vi "3dShit.vi"() -> ()   [LabVIEW 2021]
uses:
  <vilib>/Math Plots/3D Math Plots/3D Surface/3D Surface XCtrl/3D Surface.xctl
  <vilib>/Utility/file.llb/Read Delimited Spreadsheet (DBL).vi
  <vilib>/Analysis/NI_AALPro.lvlib
  <vilib>/Analysis/6fits.llb/nD B-Spline Fit.vi
  <vilib>/Math Plots/3D Math Plots/3D Surface/3D Surface Datatype/3D Surface Datatype.lvclass
  <vilib>/Math Plots/3D Math Plots/3D Surface/3D Surface Datatype/Public/Plot Helper (Matrix).vi
panel:
  in  "Slide":cluster{dbl, dbl, dbl, dbl, dbl, dbl}(slide)={248.76658476658477, 249.17936117936117, 312.74692874692875, 365.58230958230956, 381.26781326781327, 224.0} scale=224.0..392.0
  out "min value":dbl
  out "max value":dbl
  in  "Array":dbl[](array[numeric])
  out "3D Surface":refnum<class "3D Plot Datatype.lvclass">[](xcontrol)
  out "size(s)":i32[](array[numeric])
  out "Waveform Graph":dbl[][](graph)
  in  "Custom Marker Colors":u32[](array[colorbox])=[15663322, 786687, 9567230, 6618880, 16774656, 16757546, 16711680]
  in  "stop":bool
  out "Surface CV Plot":dbl[][](graph)
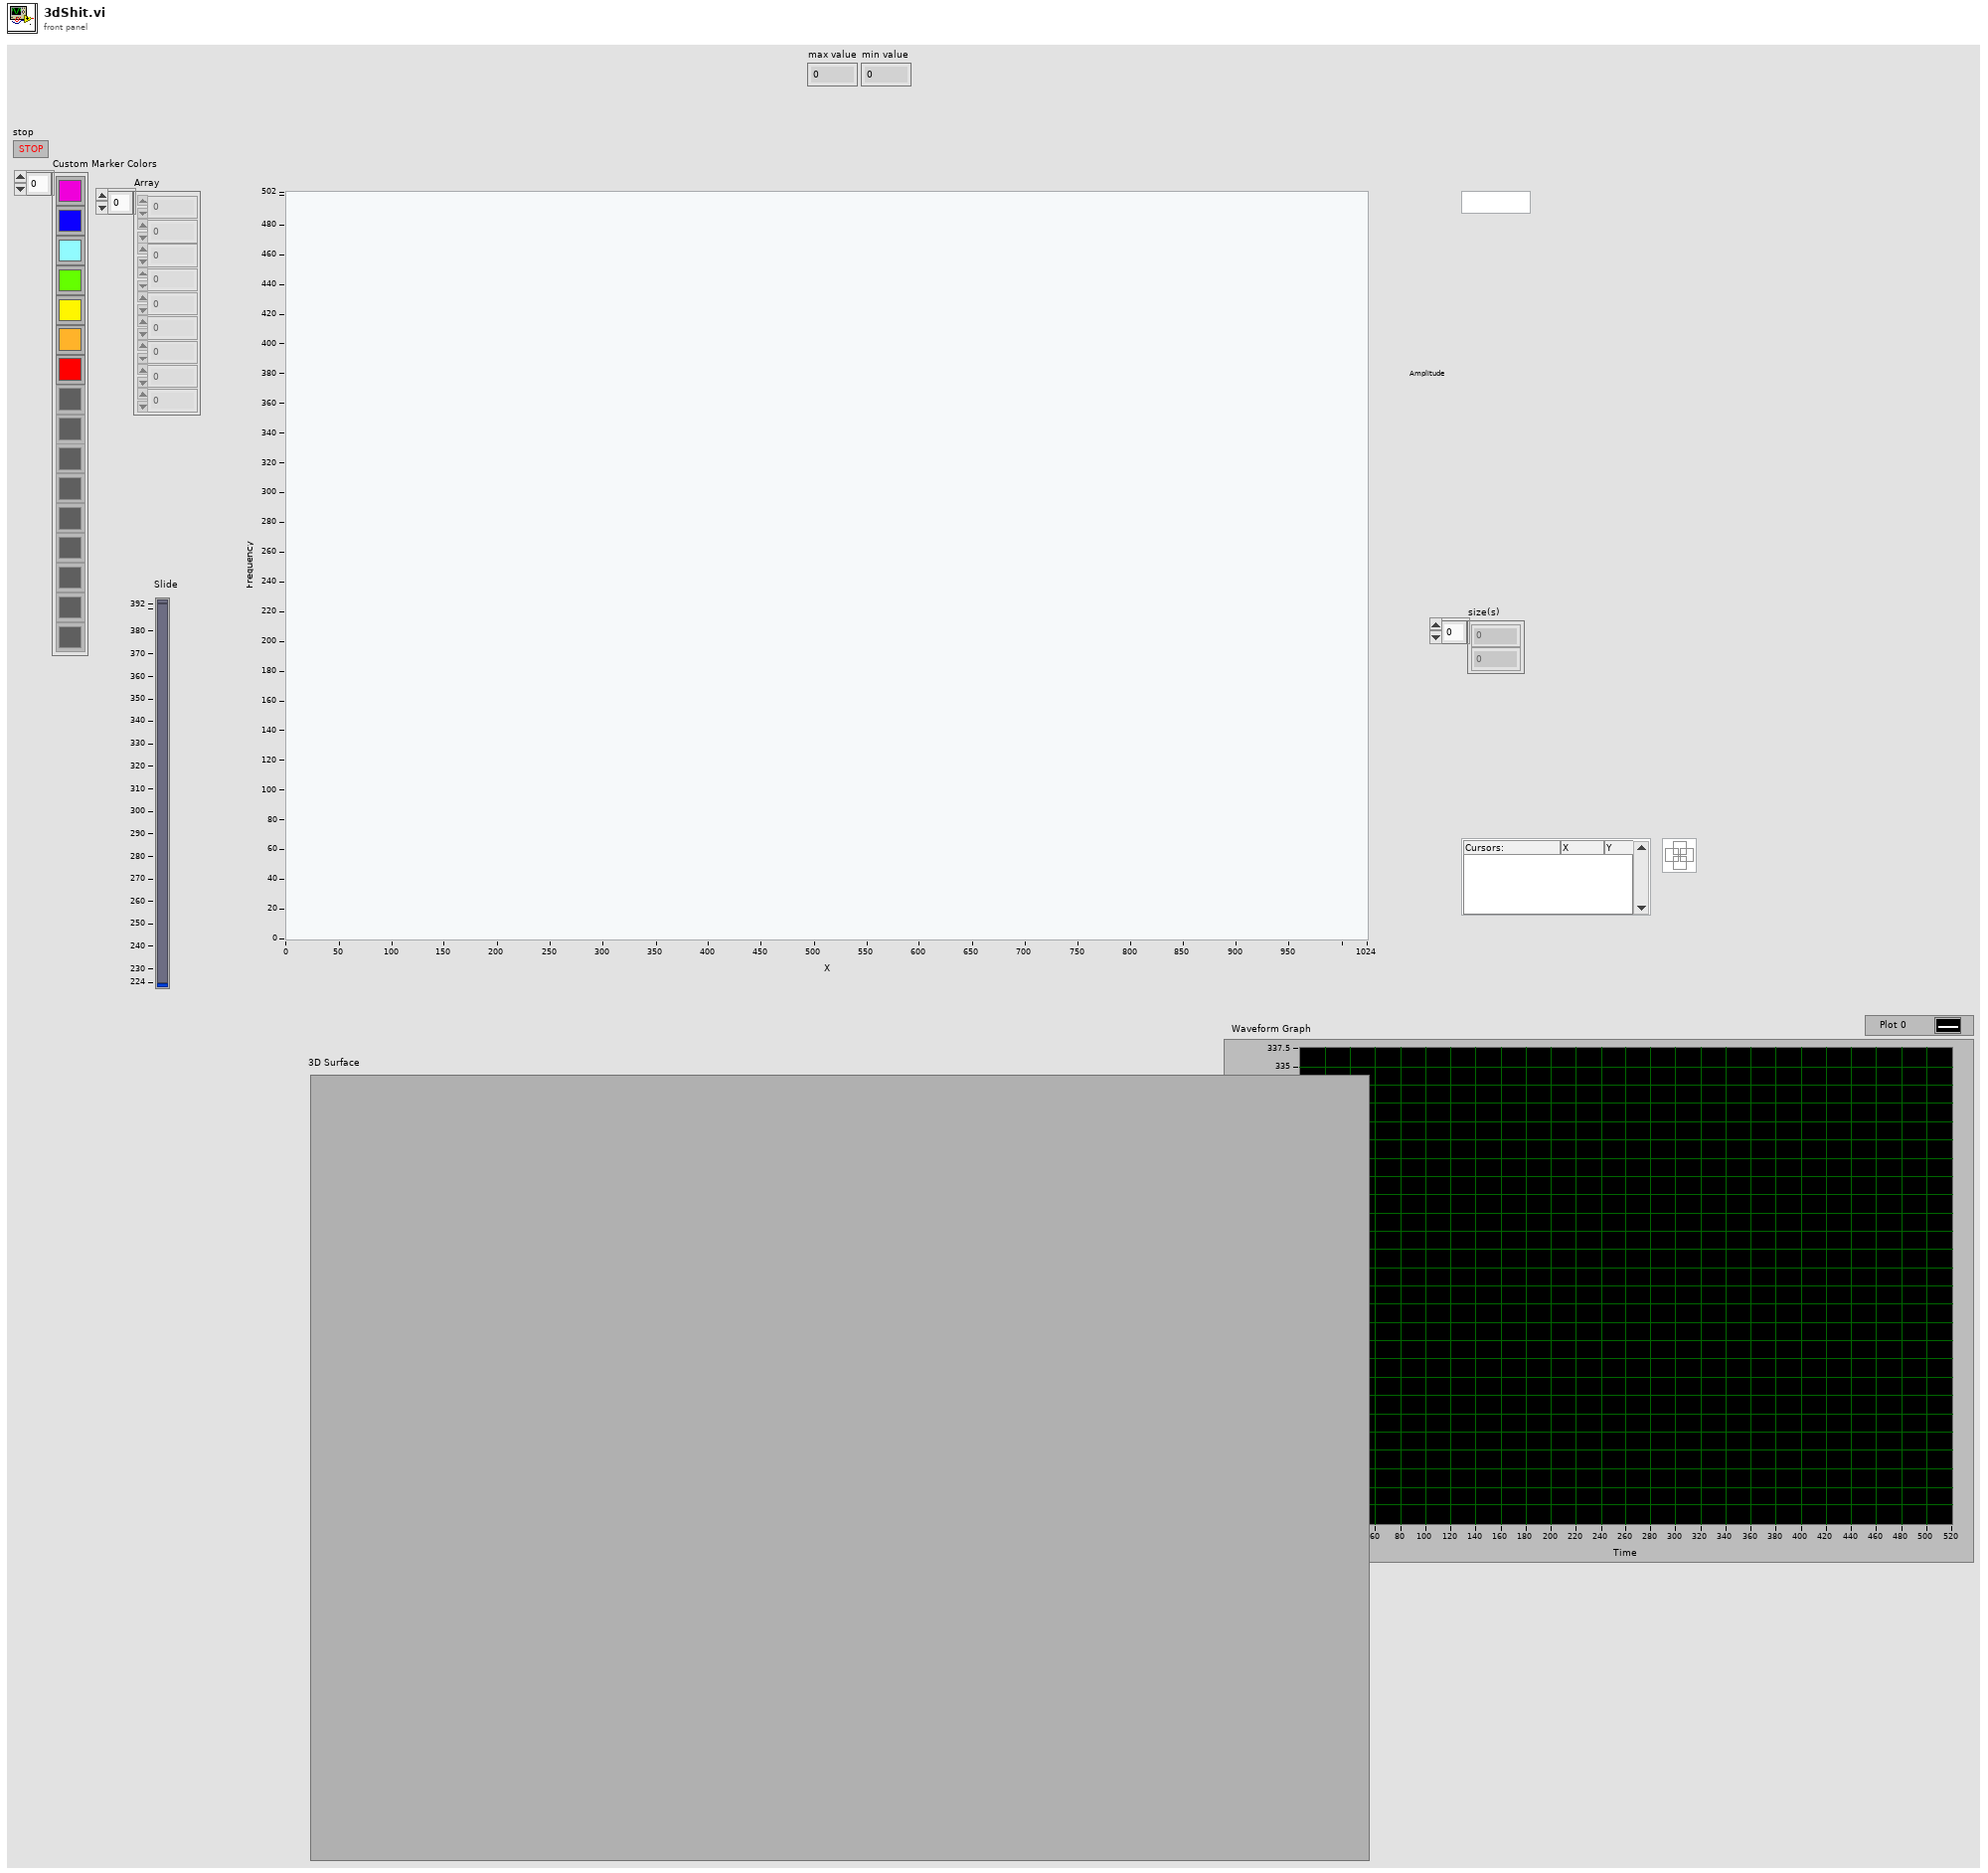
[diagram p1: front panel]
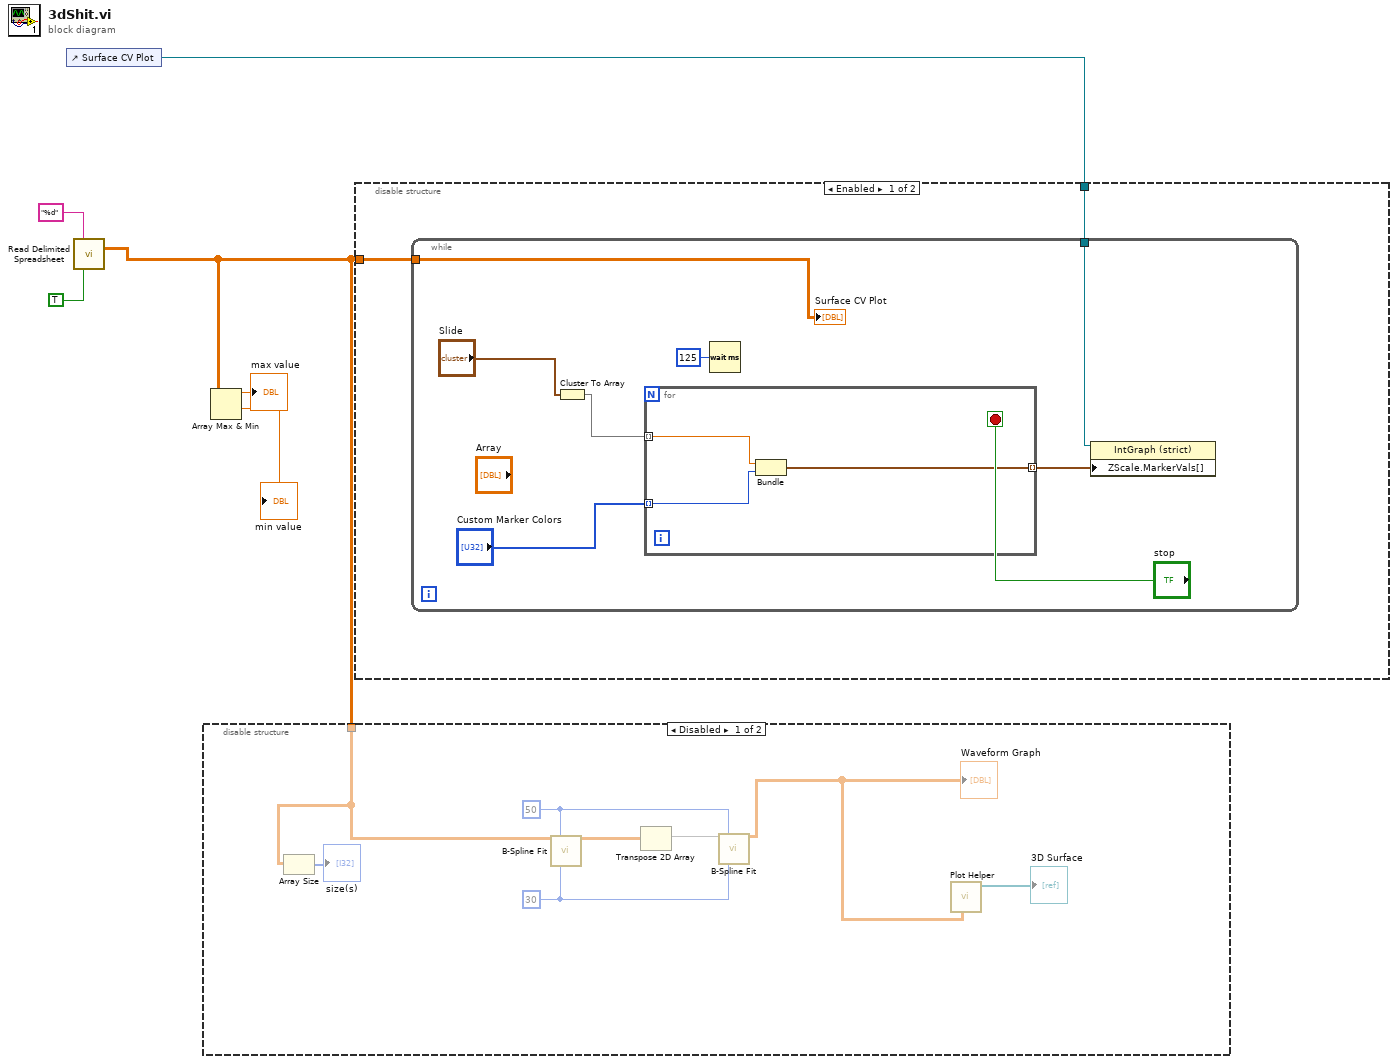
[diagram p0: block diagram]
diagram:
  n1 = control-ref of="Surface CV Plot"() -> (w4:refnum<vi>)
  n2 = call-poly <vilib>:"Read Delimited Spreadsheet.vi"("format (%.3f)"="%d", "transpose? (F)"=TRUE) -> ("all rows"=w3:dbl[][])  [unwired: 8 in, 5 out]
  n3 = disable-structure shown="Disabled" {
    disable-tunnel: w3 -> [w14 _]
    frame Disabled {
      w10 = 50 ("# of control points")
      w9 = 30 ("degree")
      n4 = Array Size(array=w14) -> (size(s)=→"size(s)":i32[])
      n5 = call-poly <vilib>:"B-Spline Fit.vi"("Data"=w14, "# of control points"=w10, "degree"=w9) -> ("Best BSpline Fit"=w12:dbl[][])  [unwired: 10 in, 2 out]
      n6 = Transpose 2D Array(2D array=w12) -> (transposed array=w11:dbl[][])
      n7 = call-poly <vilib>:"B-Spline Fit.vi"("Data"=w11, "# of control points"=w10, "degree"=w9) -> ("Best BSpline Fit"=w7:dbl[][])  [unwired: 10 in, 2 out]
      "Waveform Graph" <- w7
      n8 = call-poly <vilib>:"Plot Helper.vi"("z matrix"=w7) -> ("3D Plot lvclass Array out"=→"3D Surface":refnum<class "3D Plot Datatype.lvclass">[])  [unwired: 5 in, 5 out]
    }
    frame Enabled {
    }
  }
  n9 = Array Max & Min(array=w3) -> (max value=→"max value":dbl, min value=→"min value":dbl)  [unwired: 2 out]
  n10 = disable-structure shown="Enabled" {
    disable-tunnel: w4 -> [w16 _]
    disable-tunnel: w3 -> [w15 _]
    frame Enabled {
      n11 = while {
        tunnel: w15 -> [w24]
        tunnel: w16 -> [w19]
        stop <- "stop" stop-if-true
        n12 = Cluster To Array(cluster="Slide") -> (array=w17:dbl[])
        n13 = for {
          tunnel: "Custom Marker Colors" -> [w27] mode=indexing
          tunnel: [w26] -> w21 mode=indexing
          tunnel: w17 -> [w25] mode=indexing
          n14 = Bundle(w25, "Color Box"=w27) -> (w26:cluster{dbl, "Color Box":u32})  [unwired: 1 in]
        }
        n15 = Wait (ms)(milliseconds to wait=u32 125) -> ()  [unwired: 1 out]
        n16 = property class="IntGraph (strict)"(reference=w19, "ZScale.MarkerVals[]"=w21) -> ()  [unwired: 1 in, 2 out]
        "Surface CV Plot" <- w24
      }
    }
    frame Disabled {
    }
  }
